vi "3b. Main.vi"() -> ()   [LabVIEW 2013]
doc: "Copyright (c) 2016 Sze Howe Koh\nThis code is licensed under the MIT license"
uses:
  src/LabVIEW/LQ Core/QSize.ctl
  src/LabVIEW/Qt Widgets/QBoxLayout/Direction.ctl
  src/LabVIEW/LQ Core/LQCoreEngine/_Polymorphic Instances/Connect_EventRefOut_DBL.vi
  src/LabVIEW/Qt Widgets/QWidget/resize.vi
  src/LabVIEW/Qt Widgets/QWidget/setVisible.vi
  src/LabVIEW/LQ Core/LQCoreEngine/LQCoreEngine.lvclass
  src/LabVIEW/Qt Widgets/QLCDNumber/QLCDNumber.lvclass
  src/LabVIEW/Qwt/QwtSlider/QwtSlider.lvclass
  src/LabVIEW/Qt Widgets/QWidget/QWidget.lvclass
  src/LabVIEW/Qt Widgets/QBoxLayout/QBoxLayout.lvclass
panel:
  in  "Stop Button":bool
  # "Prerequisite knowledge/experience\n- Example 2. Managing a Widget Layout\n- Dynamically registering LabVIEW events\n\n\nDescription\nSignals are similar to Events or Notifications. Signals are handled by slots.\n\nExamples 3a, 3b and 3c show different ways of doing the same thing:  They listen for the signal that\nis emitted when you drag the slider in 2. Managing a Widget Layout, and then they use that signal\nto update the LCD.\n\nThis example uses a LabVIEW Event structure to connect the slider to the LCD.\n\n\nShowcase\n- Event-driven programming for widgets"
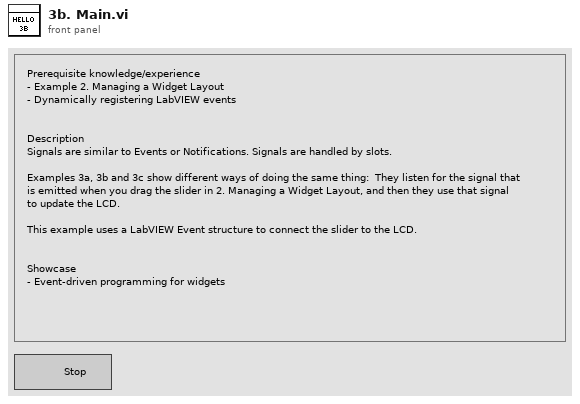
[diagram p1: front panel]
types:
  T1 = typedef "QBoxLayout.lvclass/Direction.ctl" = i32
  T2 = typedef "QSize.ctl" = cluster{"width":i32, "height":i32}
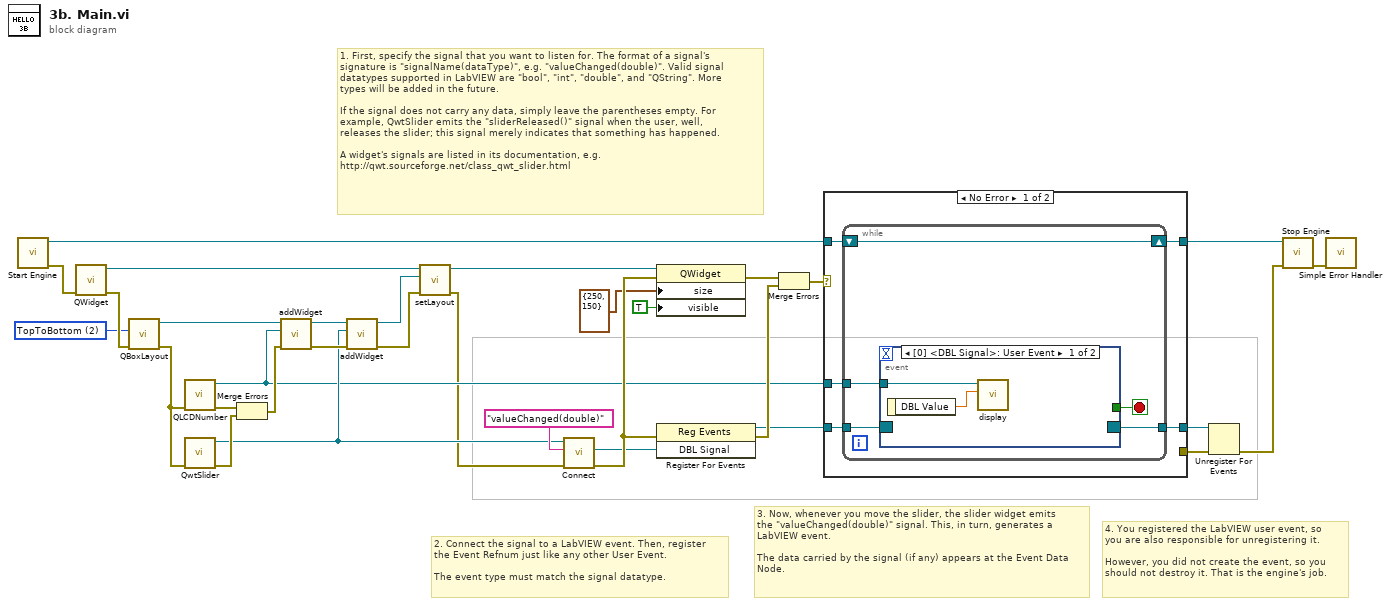
[diagram p0: block diagram]
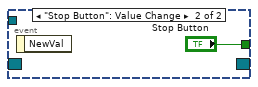
[diagram p2: hidden frame]
diagram:
  w1 = T1 2 items=["LeftToRight", "RightToLeft", "TopToBottom", "BottomToTop"] ("direction")
  # "1. First, specify the signal that you want to listen for. The format of a signal's\nsignature is \"signalName(dataType)\", e.g. \"valueChanged(double)\". Valid signal\ndatatypes supported in LabVIEW are \"bool\", \"int\", \"double\", and \"QString\". More\ntypes will be added in the future.\n\nIf the signal does not carry any data, simply leave the parentheses empty. For\nexample, QwtSlider emits the \"sliderReleased()\" signal when the user, well,\nreleases the slider; this signal merely indicates that something has happened.\n\nA widget's signals are listed in its documentation, e.g.\nhttp://qwt.sourceforge.net/class_qwt_slider.html"
  # "3. Now, whenever you move the slider, the slider widget emits\nthe \"valueChanged(double)\" signal. This, in turn, generates a\nLabVIEW event.\n\nThe data carried by the signal (if any) appears at the Event Data\nNode."
  # "2. Connect the signal to a LabVIEW event. Then, register\nthe Event Refnum just like any other User Event.\n\nThe event type must match the signal datatype."
  # "4. You registered the LabVIEW user event, so\nyou are also responsible for unregistering it.\n\nHowever, you did not create the event, so you\nshould not destroy it. That is the engine's job."
  n1 = call "Start Engine.vi"() -> ("Error Out"=w17:errorcluster, "New Engine"=w6:refnum<class "LQCoreEngine.lvclass">)  [unwired: 10 in]
  n2 = call "QWidget.vi"("Error In"=w17) -> ("Error Out"=w16:errorcluster, "New QWidget"=w9:refnum<class "QWidget.lvclass">)  [unwired: 9 in]
  n3 = call "QBoxLayout.vi"("Error In"=w16, "direction"=w1) -> ("Error Out"=w15:errorcluster, "New QBoxLayout"=w14:refnum<class "QBoxLayout.lvclass">)  [unwired: 8 in]
  n4 = call "QLCDNumber.vi"("Error In"=w15) -> ("Error Out"=w12:errorcluster, "New QLCDNumber"=w3:refnum<class "QLCDNumber.lvclass">)  [unwired: 9 in]
  n5 = call "QwtSlider.vi"("Error In"=w15) -> ("Error Out"=w13:errorcluster, "New QwtSlider"=w5:refnum<class "QwtSlider.lvclass">)  [unwired: 9 in]
  n6 = Merge Errors(w12, w13) -> (w18:errorcluster)
  n7 = call "addWidget.vi"("Error In"=w18, "widget"=w3, "QBoxLayout In"=w14) -> ("Error Out"=w10:errorcluster, "QBoxLayout Out"=w11:refnum<class "QBoxLayout.lvclass">)  [unwired: 7 in]
  n8 = call "addWidget.vi"("Error In"=w10, "widget"=w5, "QBoxLayout In"=w11) -> ("Error Out"=w7:errorcluster, "QBoxLayout Out"=w8:refnum<class "QBoxLayout.lvclass">)  [unwired: 7 in]
  n9 = call "setLayout.vi"("Error In"=w7, "layout"=w8, "QWidget In"=w9) -> ("Error Out"=w2:errorcluster, "QWidget Out"=w4:refnum<class "QWidget.lvclass">)  [unwired: 7 in]
  n10 = call-poly "Connect.vi"("Error In"=w2, "Signal Signature"="valueChanged(double)", "Sender In"=w5) -> ("Error Out"=w31:errorcluster, "DBL Signal"=w24:refnum<user-event>)  [unwired: 6 in, 1 out]
  n11 = property class="QWidget"(reference=w4, error in=w31, "size"=T2 {"width"=250, "height"=150}, "visible"=TRUE) -> (error out=w28:errorcluster)  [unwired: 1 out]
  n12 = register-events(error in=w31, w24) -> (reference out=w23:refnum<event-registration>, error out=w32:errorcluster)  [unwired: 1 in]
  n13 = Merge Errors(w28, w32) -> (w20:errorcluster)
  n14 = case shown="No Error" w20 {
    selector: w20 -> [_ w46]
    tunnel: w6 -> [w37 w48]
    tunnel: [w36 w48] -> w29
    tunnel: w23 -> [w35 w47]
    tunnel: [w34 w47] -> w22
    tunnel: [_ w46] -> w19
    tunnel: w3 -> [w33 _]
    frame No Error {
      n15 = while {
        shift-right: [w42] -> w36
        shift-left: w37 -> [w42]
        tunnel: w35 -> [w41]
        tunnel: [w39] -> w34
        tunnel: w33 -> [w38]
        stop <- w40 stop-if-true
        n16 = event shown="[0] <DBL Signal>: User Event" {
          selector: w41 -> [_ _]
          dyn-events: [_ _] -> w39
          timeout: _ -> [_ _]
          tunnel: [_ "Stop Button"] -> w40
          tunnel: w38 -> [w44 _]
          event User Event {
            n17 = event-data() -> ("DBL Value"=w43:dbl)  [unwired: 1 in]
            n18 = call "display.vi"("num"=w43, "QLCDNumber In"=w44) -> ()  [unwired: 8 in, 2 out]
          }
          event "Stop Button": Value Change {
            n19 = event-data() -> ()  [unwired: 1 in, 1 out]
          }
        }
      }
    }
    frame Error {
    }
  }
  n20 = Unregister For Events(event registration refnum=w22, error in=w19) -> (error out=w21:errorcluster)
  n21 = call "Stop Engine.vi"("Error In"=w21, "LQCoreEngine"=w29) -> ("Error Out"=w27:errorcluster)  [unwired: 9 in]
  n22 = call <vilib>:"Simple Error Handler.vi"("error in (no error)"=w27) -> ()  [unwired: 4 in, 5 out]
